vi "PADMINI_BOOL_COLOR_CHANGE.vi"(8 "error in (no error)":errorcluster, 10 "Numeric":u16, 11 "Boolean in":refnum<vi>) -> (0 "error out":errorcluster)   [LabVIEW 2023]
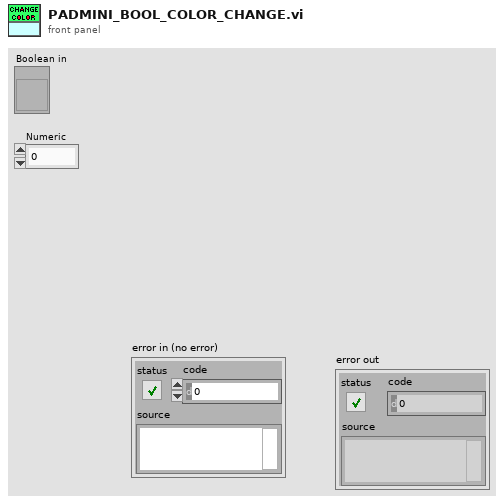
[diagram p1: front panel]
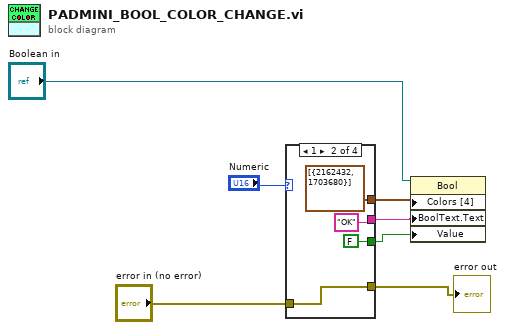
[diagram p0: block diagram]
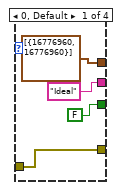
[diagram p2: hidden frame]
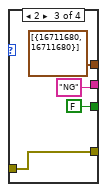
[diagram p3: hidden frame]
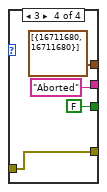
[diagram p4: hidden frame]
diagram:
  n1 = case shown="1" "Numeric" {
    tunnel: [cluster{u32, u32}[] [{16776960, 16776960}] ("Colors [4]") cluster{u32, u32}[] [{2162432, 1703680}] ("Colors [4]") cluster{u32, u32}[] [{16711680, 16711680}] ("Colors [4]") cluster{u32, u32}[] [{16711680, 16711680}] ("Colors [4]")] -> w5
    tunnel: ["Ideal" "OK" "NG" "Aborted"] -> w6
    tunnel: [FALSE FALSE FALSE FALSE] -> w1
    tunnel: [w8 w12 w16 w20] -> w3
    tunnel: "error in (no error)" -> [w8 w12 w16 w20]
    frame 0, Default {
    }
    frame 1 {
    }
    frame 2 {
    }
    frame 3 {
    }
  }
  "error out" <- w3
  n2 = property on="Property Node" class="Bool"(reference="Boolean in", "Colors [4]"=w5, "BoolText.Text"=w6, "Value"=w1) -> ()  [unwired: 1 in, 2 out]
